vi "Scalar Data to String.vi"(11 "Data":variant) -> (0 "error out":errorcluster, 2 "Value String":string)   [LabVIEW 2020, in "VariantExtensions.lvlib"]
doc: "标量数据到字符串"
uses:
  VariantExtensions.lvlib
  <vilib>/Utility/Data Type/NI_Data Type.lvlib
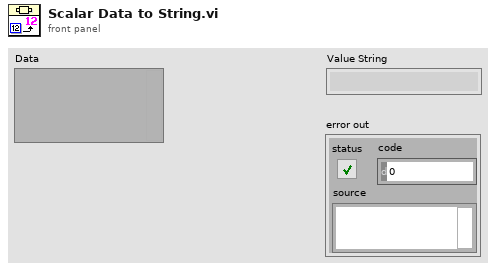
[diagram p1: front panel]
types:
  T1 = typedef "NI_Data Type.lvlib/Data Type.ctl" = enum8{"Invalid Type", "Void", "I8", "I16", "I32", "I64", "U8", "U16", "U32", "U64", "Single Float", "Double Float", "Extended Float", "Single Complex", "Double Complex", "Extended Complex", "Enum U8", "Enum U16", "Enum U32", "Enum U64", "Single Float With Unit", "Double Float With Unit", "Extended Float With Unit", "Single Complex with Unit", "Double Complex with Unit", "Extended Complex with Unit", "Boolean", "String", "Path", "Picture", "Tag", "Array", "Cluster", "Variant", "LV Variant", "Waveform", "Timestamp", "Digital Waveform", "Digital Data", "ExpressData", "Refnum", "External Data", "VI", "Poly VI", "LabVIEW Class Instance", "Fixed Point", "Set Collection", "Map Collection"}
  T2 = typedef "NI_Data Type.lvlib/Refnum Type.ctl" = enum16{"NotARefnum", "UnknownRefnum", "Generic", "Datalog", "ByteStream", "Device", "Occurence", "TCPNetConnection", "Auto", "Menu", "Imaq", "Hardware", "DataSocket", "Visa", "IVI", "UDPNetConnection", "Notifier", "Queue", "Irda", "EventReg", "DotNet", "UserEvent", "Callback", "UNUSED_EMPTY_POSITION", "BlueToothNetConnection", "LVObjApp", "LVObjVI", "LVObjUnknown", "GenericClass", "UserDefinedRefnumTag", "DataValue", "RT FIFO", "TDMS File", "PythonSessionRefnum"}
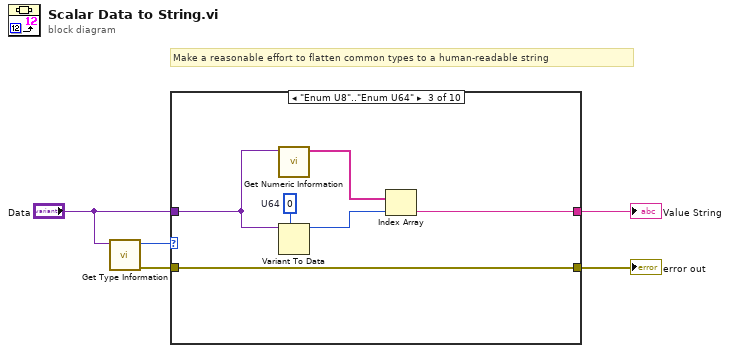
[diagram p0: block diagram]
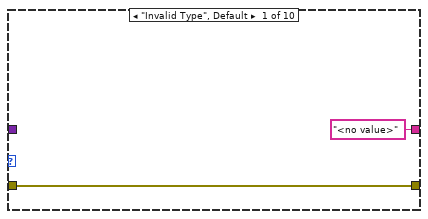
[diagram p2: hidden frame]
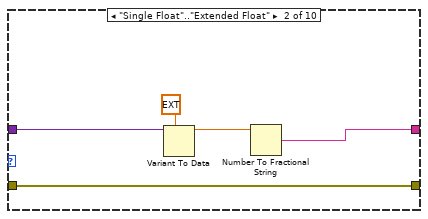
[diagram p3: hidden frame]
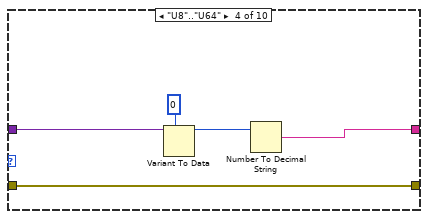
[diagram p4: hidden frame]
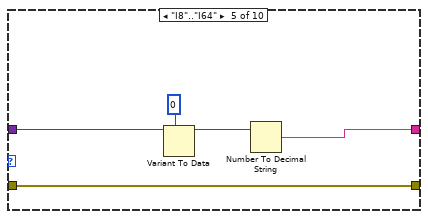
[diagram p5: hidden frame]
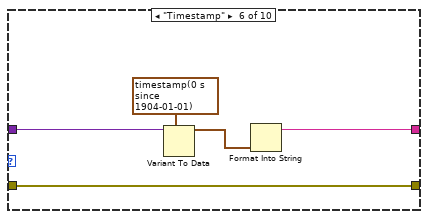
[diagram p6: hidden frame]
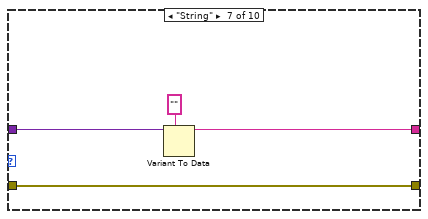
[diagram p7: hidden frame]
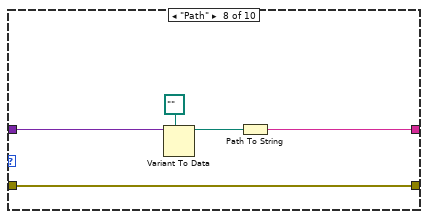
[diagram p8: hidden frame]
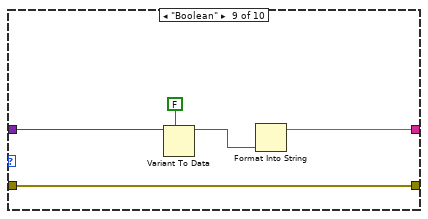
[diagram p9: hidden frame]
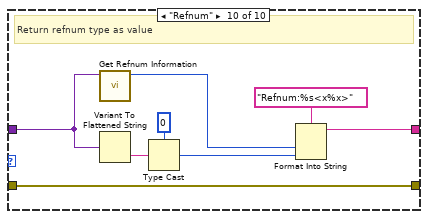
[diagram p10: hidden frame]
diagram:
  # "Make a reasonable effort to flatten common types to a human-readable string"
  n1 = call <vilib>:"Get Type Information.vi"("variant"="Data") -> ("error out"=w3:errorcluster, "type"=w2:T1)  [unwired: 6 in, 3 out]
  n2 = case shown="\"Enum U8\"..\"Enum U64\"" w2 {
    tunnel: "Data" -> [_ w11 w16 w22 w27 w32 w36 w41 w46 w51]
    tunnel: ["<no value>" w10 w17 w21 w26 w29 w35 w39 w43 w53] -> w4
    tunnel: w3 -> [w7 w8 w18 w19 w24 w31 w34 w38 w45 w55]
    tunnel: [w7 w8 w18 w19 w24 w31 w34 w38 w45 w55] -> w1
    frame "Invalid Type", Default {
    }
    frame "Single Float".."Extended Float" {
      n3 = Variant To Data(type=ext 0.0, Variant=w11) -> (data=w9:ext)  [unwired: 1 in, 1 out]
      n4 = Number To Fractional String(number=w9) -> (F-format string=w10:string)  [unwired: 3 in]
    }
    frame "Enum U8".."Enum U64" {
      w15 = u64 0  # U64
      n5 = call <vilib>:"Get Numeric Information.vi"("variant"=w16) -> ("enum names"=w14:string[])  [unwired: 7 in, 3 out]
      n6 = Variant To Data(type=w15, Variant=w16) -> (data=w13:u64)  [unwired: 1 in, 1 out]
      n7 = Index Array(array=w14, index=w13) -> (element=w17:string)
    }
    frame "U8".."U64" {
      n8 = Variant To Data(type=u64 0, Variant=w22) -> (data=w20:u64)  [unwired: 1 in, 1 out]
      n9 = Number To Decimal String(number=w20) -> (decimal integer string=w21:string)  [unwired: 1 in]
    }
    frame "I8".."I64" {
      n10 = Variant To Data(type=i64 0, Variant=w27) -> (data=w25:i64)  [unwired: 1 in, 1 out]
      n11 = Number To Decimal String(number=w25) -> (decimal integer string=w26:string)  [unwired: 1 in]
    }
    frame "Timestamp" {
      n12 = Variant To Data(type=timestamp(0 s since 1904-01-01), Variant=w32) -> (data=w30:timestamp)  [unwired: 1 in, 1 out]
      n13 = Format Into String(w30) -> (resulting string=w29:string)  [unwired: 3 in, 1 out]
    }
    frame "String" {
      n14 = Variant To Data(type="", Variant=w36) -> (data=w35:string)  [unwired: 1 in, 1 out]
    }
    frame "Path" {
      n15 = Variant To Data(type=path "", Variant=w41) -> (data=w40:path)  [unwired: 1 in, 1 out]
      n16 = Path To String(path=w40) -> (string=w39:string)
    }
    frame "Boolean" {
      n17 = Variant To Data(type=FALSE, Variant=w46) -> (data=w44:bool)  [unwired: 1 in, 1 out]
      n18 = Format Into String(w44) -> (resulting string=w43:string)  [unwired: 3 in, 1 out]
    }
    frame "Refnum" {
      # "Return refnum type as value"
      n19 = call <vilib>:"Get Refnum Information.vi"("variant"=w51) -> ("reference type"=w54:T2)  [unwired: 7 in, 3 out]
      n20 = Variant To Flattened String(Variant=w51) -> (data string=w50:string)  [unwired: 1 out]
      n21 = Type Cast(type=u32 0, x=w50) -> (*(type *) &x=w48:u32)
      n22 = Format Into String(format string="Refnum:%s<x%x>", w54, w48) -> (resulting string=w53:string)  [unwired: 2 in, 1 out]
    }
  }
  "error out" <- w1
  "Value String" <- w4
